vi "Log Data.vi"(8 "error in (no error)":errorcluster, 10 "Data Queue":T1, 11 "Logging Configuration":T2) -> (0 "error out":errorcluster)   [LabVIEW 2015, in "Logging.lvlib"]
doc: "This VI uses the TDMS Write function to write data to a TDMS file."
uses:
  Logging.lvlib
  Logging Configuration.ctl
  controls/Data queue.ctl
  Acquisition/Generic data packet.ctl
  My Graphs/Gps Map Graph coordinates.ctl
  Acquisition/Acquisition.lvlib
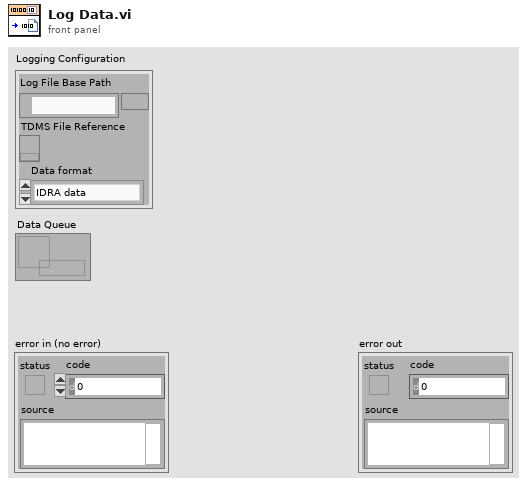
[diagram p1: front panel]
types:
  T1 = typedef "Data queue.ctl" = refnum<queue>
  T2 = typedef "Logging.lvlib/Logging Configuration.ctl" = cluster{"Log File Base Path":path, "TDMS File Reference":refnum<k34>, "Data format":enum16{"IDRA data", "XAM data"}}
  T3 = typedef "Acquisition.lvlib/Generic data packet.ctl" = cluster{"Content type":enum16{"None", "Telemetria", "GPS"}, "GPS":T4, "Telemetria":cluster{"Data format":enum16{"IDRA data", "XAM data"}, "Data":variant}}
  T4 = typedef "Gps Map Graph coordinates.ctl" = cluster{"Latitude":dbl, "Longitude":dbl}
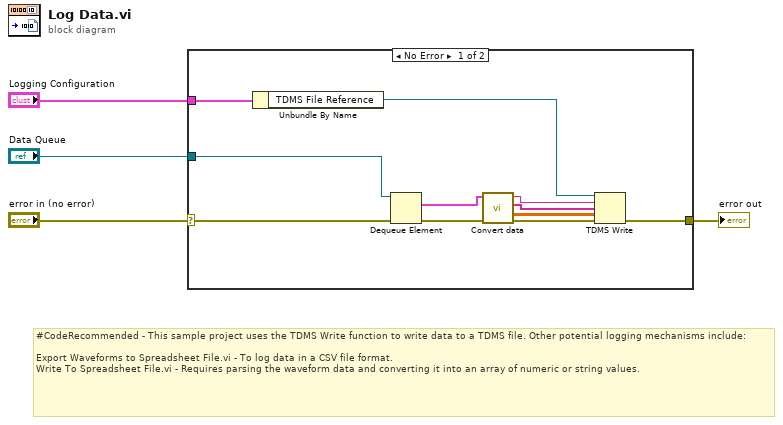
[diagram p0: block diagram]
diagram:
  # "#CodeRecommended - This sample project uses the TDMS Write function to write data to a TDMS file. Other potential logging mechanisms include:\n\nExport Waveforms to Spreadsheet File.vi - To log data in a CSV file format.\nWrite To Spreadsheet File.vi - Requires parsing the waveform data and converting it into an array of numeric or string values."
  n1 = case shown="No Error" "error in (no error)" {
    selector: "error in (no error)" -> [w13 w16]
    tunnel: "Logging Configuration" -> [w15 _]
    tunnel: "Data Queue" -> [w12 _]
    tunnel: [w14 w16] -> w2
    frame No Error {
      n2 = Unbundle By Name(w15) -> ("TDMS File Reference"=w11:refnum<k34>)
      n3 = Dequeue Element(queue=w12, error in (no error)=w13) -> (element=w8:T3, error out=w10:errorcluster)  [unwired: 1 in, 2 out]
      n4 = call "Convert data.vi"("Error in"=w10, "Element in"=w8) -> ("Error out"=w9:errorcluster, "Data out"=w5:dbl[][], "Channels name"=w6:string[], "Content type"=w7:string)  [unwired: 6 in]
      n5 = TDMS Write(0:w11, 5:w7, 7:w6, 9:w5, 11:w9) -> (15:w14:errorcluster)  [unwired: 1 in, 3 out]
    }
    frame Error {
    }
  }
  "error out" <- w2
